vi "Read Data.vi"(8 "error in (no error)":errorcluster caption="错误输入（无错误）", 11 "HL7 输入":refnum<class "HL7.lvclass">) -> (0 "error out":errorcluster caption="错误输出", 3 "HL7 输出":refnum<class "HL7.lvclass">)   [LabVIEW 2016, in "HL7.lvlib" / "HL7.lvclass"]
uses:
  HL7.lvclass
  <vilib>/Plasmionique/MB Master/MB Master.lvlib
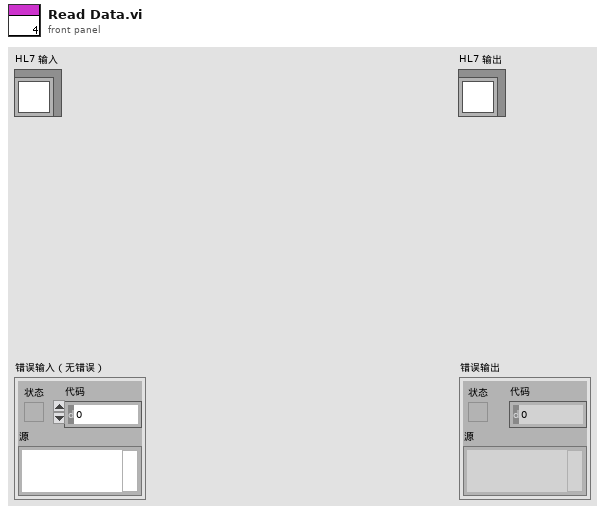
[diagram p1: front panel]
types:
  T1 = cluster{"[0]":sgl, "[1]":sgl, "[2]":sgl, "[3]":sgl, "[4]":sgl, "[5]":sgl, "[6]":sgl, "[7]":sgl, "[8]":sgl, "[9]":sgl}
  T2 = cluster{"Time":timestamp, "Temp":dbl, "SpCond":dbl, "Cond":dbl, "Sal":dbl, "TDS":dbl, "pH":dbl, "pH mV":dbl, "orp":dbl, "ODO %":dbl, "ODO mg/L":dbl, "Turb":dbl, "Chl":dbl, "BGA":dbl, "Depth":dbl}
  T3 = cluster{"水温":sgl, "比电导率_mS/cm":sgl, "DO%":sgl, "DO_mg/L":sgl, "pH":sgl, "depth_m":sgl, "盐度_psu":sgl, "浊度_NTU":sgl, "叶绿素a_μg/L":sgl, "电导率_μS/cm":sgl}
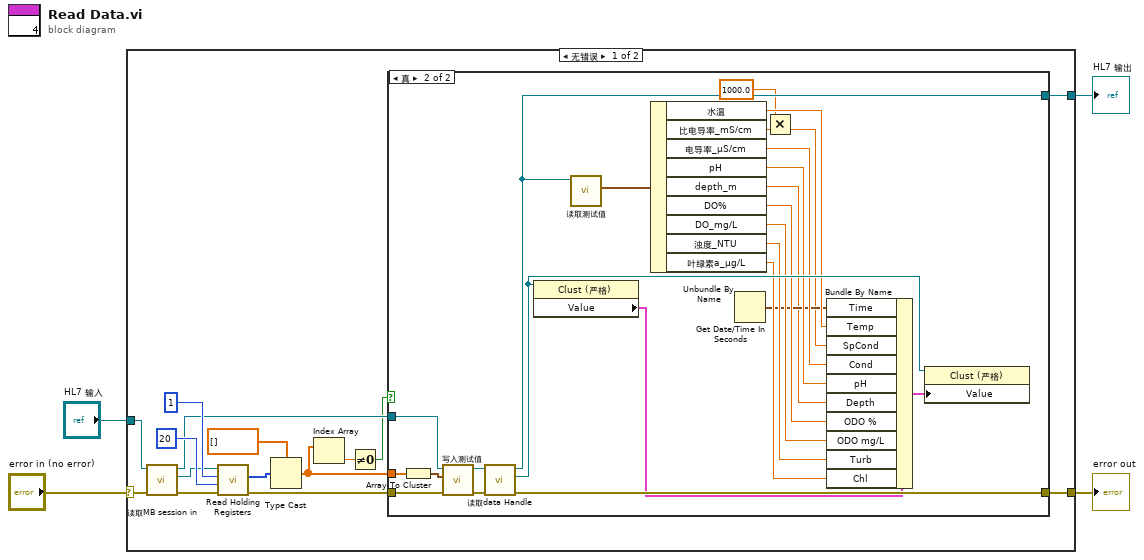
[diagram p0: block diagram]
diagram:
  n1 = case shown="无错误" "error in (no error)" {
    selector: "error in (no error)" -> [w11 w47]
    tunnel: [w5 w47] -> w3
    tunnel: [w8 w46] -> w1
    tunnel: "HL7 输入" -> [w19 w46]
    frame No Error {
      n2 = call-dynamic "读取MB session in.vi"("error in (no error)"=w11, "HL7输入"=w19) -> ("error out"=w12:errorcluster, "MB Serial Master:MB_Master"=w13:refnum<class "MB_Master.lvclass">, "HL7输出"=w9:refnum<class "HL7.lvclass">)  [unwired: 7 in]
      n3 = call <vilib>:"Read Holding Registers.vi"("error in (no error)"=w12, "quantity"=u16 20, "starting address"=u16 1, "MB session in"=w13) -> ("error out"=w6:errorcluster, "Registers"=w16:u16[])  [unwired: 5 in, 1 out]
      n4 = Type Cast(type=sgl[] [], x=w16) -> (*(type *) &x=w10:sgl[])
      n5 = Index Array(array=w10) -> (element=w14:sgl)  [unwired: 1 in]
      n6 = Not Equal To 0?(x=w14) -> (x != 0?=w7:bool)
      n7 = case shown="真" w7 {
        tunnel: w10 -> [_ w45]
        tunnel: w9 -> [w21 w44]
        tunnel: [w21 w37] -> w8
        tunnel: w6 -> [w20 w43]
        tunnel: [w20 w39] -> w5
        frame False {
        }
        frame True {
          n8 = Array To Cluster(array=w45) -> (cluster=w40:T1)
          n9 = call-dynamic "写入测试值.vi"("error in (no error)"=w43, "测试值"=w40, "HL7输入"=w44) -> ("error out"=w41:errorcluster, "HL7输出"=w42:refnum<class "HL7.lvclass">)  [unwired: 7 in]
          n10 = call-dynamic "读取data Handle.vi"("error in (no error)"=w41, "HL7输入"=w42) -> ("error out"=w39:errorcluster, "data Handle"=w38:refnum<vi>, "HL7输出"=w37:refnum<class "HL7.lvclass">)  [unwired: 7 in]
          n11 = property class="Clust (严格)"(reference=w38) -> ("Value"=w35:T2)  [unwired: 1 in, 2 out]
          n12 = call-dynamic "读取测试值.vi"("HL7输入"=w37) -> ("测试值"=w36:T3)  [unwired: 8 in, 2 out]
          n13 = Unbundle By Name(w36) -> ("水温"=w34:sgl, "比电导率_mS/cm"=w33:sgl, "电导率_μS/cm"=w32:sgl, "pH"=w31:sgl, "depth_m"=w24:sgl, "DO%"=w30:sgl, "DO_mg/L"=w29:sgl, "浊度_NTU"=w28:sgl, "叶绿素a_μg/L"=w27:sgl)
          n14 = Get Date/Time In Seconds() -> (seconds since 1Jan1904=w26:timestamp)
          n15 = Multiply(x=sgl 1000.0, y=w33) -> (x*y=w23:sgl)
          n16 = Bundle By Name(cluster=w35, "Time"=w26, "Temp"=w34, "SpCond"=w23, "Cond"=w32, "pH"=w31, "Depth"=w24, "ODO %"=w30, "ODO mg/L"=w29, "Turb"=w28, "Chl"=w27) -> (w25:T2)
          n17 = property class="Clust (严格)"(reference=w38, "Value"=w25) -> ()  [unwired: 1 in, 2 out]
        }
      }
    }
    frame Error {
    }
  }
  "error out" <- w3
  "HL7 输出" <- w1
